vi "Reorder VI info.vi"(1 "chain":string) -> (0 "Reorderded":string)   [LabVIEW 2011, in "Messenging.lvlib" / "Message Logger.lvclass"]
uses:
  Message Logger.lvclass
  <vilib>/regexp/Match Regular Expression.xnode
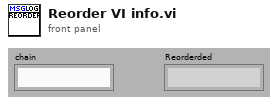
[diagram p1: front panel]
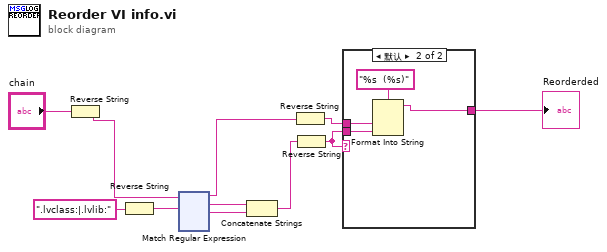
[diagram p0: block diagram]
diagram:
  n1 = Reverse String(1:"chain") -> (0:w8:string)
  n2 = Reverse String(1:".lvclass:|.lvlib:" ("regular expression")) -> (0:w6:string)
  n3 = xnode "Match Regular Expression"("输入字符串"=w8, "正则表达式"=w6) -> ("匹配之前"=w5:string, "所有匹配"=w2:string, "匹配之后"=w4:string)  [unwired: 2 in, 4 out]
  n4 = Concatenate Strings(w2, w4) -> (w3:string)
  n5 = Reverse String(1:w5) -> (0:w10:string)
  n6 = Reverse String(1:w3) -> (0:w1:string)
  n7 = case shown="默认" w1 {
    tunnel: w10 -> [w12 w15]
    tunnel: w1 -> [_ w14]
    tunnel: [w12 w13] -> w9
    frame "" {
    }
    frame Default {
      n8 = Format Into String(format string="%s  (%s)", w15, w14) -> (resulting string=w13:string)  [unwired: 2 in, 1 out]
    }
  }
  "Reorderded" <- w9
